vi "CRYUnflatten Work State.vi"(11 "Unflatten work state #":string) -> (0 "Error?":bool=TRUE, 3 "Header info":T1={"Data type"="Data            ", "Version"=1, "Dimensions"=0})   [LabVIEW 2013]
uses:
  CRYSystem/Hardware/CRYHardware Global.vi
  CRYSystem/Calibration/SubVI/CRYCal Global.vi
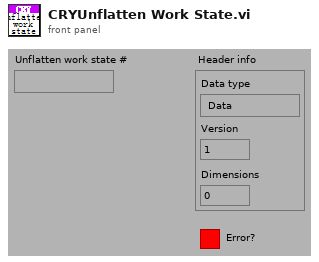
[diagram p1: front panel]
types:
  T1 = cluster{"Data type":string, "Version":u16, "Dimensions":u8}
  T2 = cluster{"unsigned byte array[0]":u8, "unsigned byte array[1]":u8, "unsigned byte array[2]":u8}
  T3 = cluster{"Mic Vol-L":dbl, "Mic Vol-R":dbl, "Mic Res-L":dbl, "Mic Res-R":dbl}
  T4 = cluster{"Mic Vol-L":dbl, "Mic Vol-R":dbl, "Mic Res-L":dbl, "Mic Res-R":dbl, "Mic Res-R 2":dbl, "Mic Res-R 3":dbl}
  T5 = cluster{"substring":string, u16, "unsigned byte array[2]":u8}
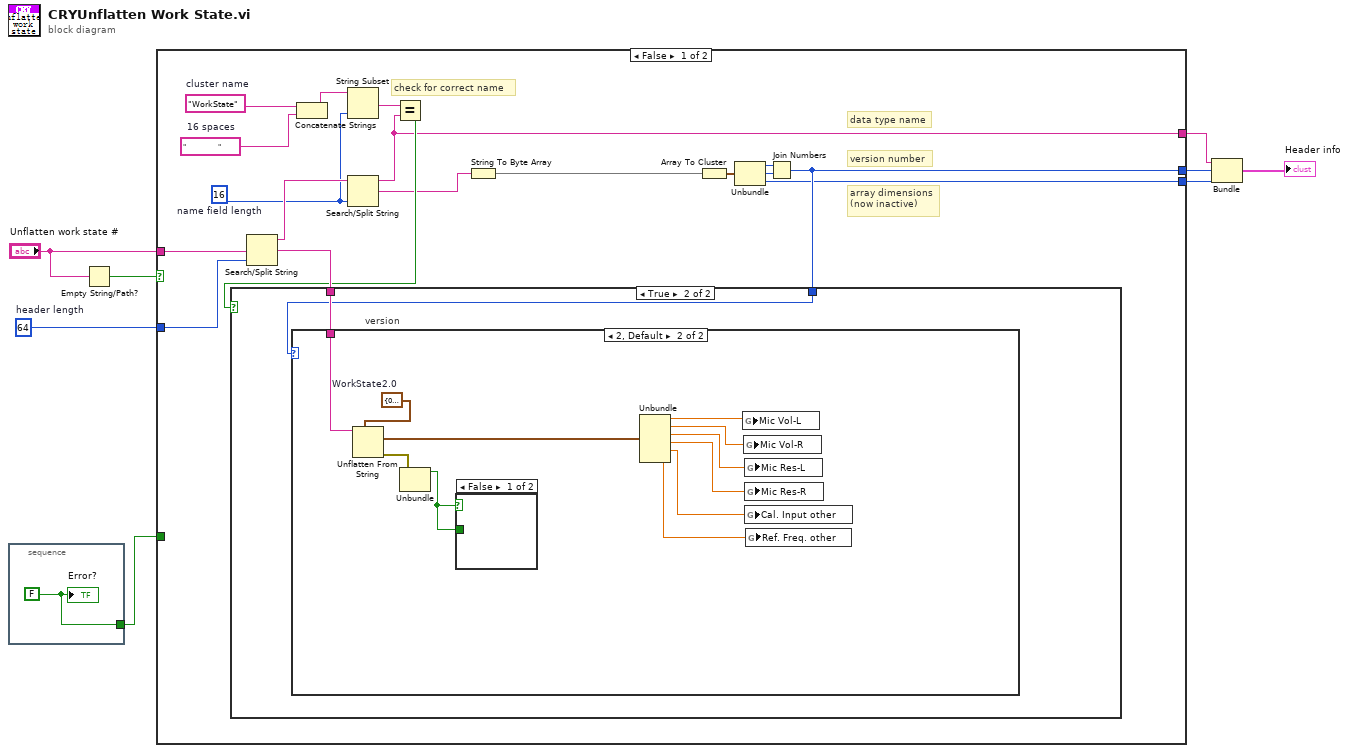
[diagram p0: block diagram]
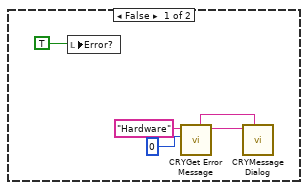
[diagram p2: hidden frame]
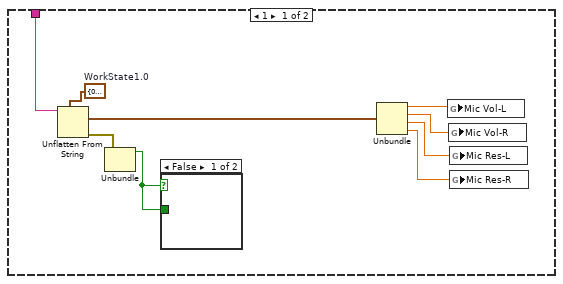
[diagram p3: hidden frame]
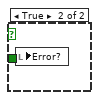
[diagram p4: hidden frame]
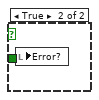
[diagram p5: hidden frame]
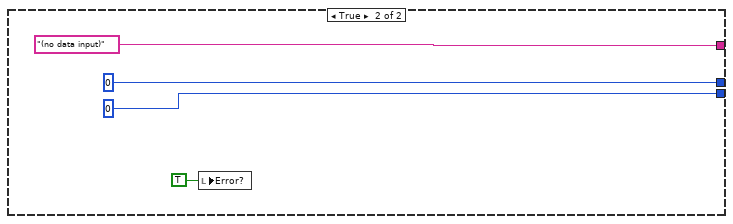
[diagram p6: hidden frame]
diagram:
  w5 = 64  # header length
  n1 = stacked-sequence {
    tunnel: [w9] -> w1
    frame #0 {
      w9 = FALSE
      "Error?" <- w9
    }
  }
  n2 = Empty String/Path?(string/path="Unflatten work state #") -> (empty?=w6:bool)
  n3 = case shown="False" w6 {
    tunnel: "Unflatten work state #" -> [w27 _]
    tunnel: w5 -> [w21 _]
    tunnel: [w18 u16 0] -> w3
    tunnel: [w10 u8 0] -> w4
    tunnel: [w11 "(no data input)" ("substring")] -> w2
    tunnel: w1 -> [_ _]
    frame False {
      w15 = "                "  # 16 spaces
      w16 = "WorkState"  # cluster name
      w13 = 16  # name field length
      # "check for correct name"
      # "array dimensions\n(now inactive)"
      # "version number"
      # "data type name"
      n4 = Search/Split String(string=w27, offset (0)=w21) -> (substring before match=w20:string, match + rest of string=w22:string)  [unwired: 2 out]
      n5 = Concatenate Strings(w16, w15) -> (w14:string)
      n6 = String Subset(string=w14, length (rest)=w13) -> (substring=w12:string)  [unwired: 1 out]
      n7 = Search/Split String(string=w20, offset (0)=w13) -> (substring before match=w11:string, match + rest of string=w17:string)  [unwired: 2 out]
      n8 = Equal?(x=w12, y=w11) -> (x = y?=w19:bool)
      n9 = String To Byte Array(string=w17) -> (unsigned byte array=w26:u8[])
      n10 = Array To Cluster(array=w26) -> (cluster=w25:T2)
      n11 = Unbundle(w25) -> ("unsigned byte array[0]"=w24:u8, "unsigned byte array[1]"=w23:u8, "unsigned byte array[2]"=w10:u8)
      n12 = Join Numbers(hi=w24, lo=w23) -> ((hi.lo)=w18:u16)
      n13 = case shown="True" w19 {
        tunnel: w22 -> [_ w34]
        tunnel: w18 -> [_ w33]
        frame False {
          n14 = local write "Error?"(TRUE) -> ()
          n15 = call "CRYGet Error Message.vi"("Error No"=0, "Kind"="Hardware") -> ("Message"=w29:string, "Window Title"=w28:string)  [unwired: 4 in, 4 out]
          n16 = call "CRYMessage Dialog.vi"("Window Title"=w28, "Message Content"=w29) -> ()  [unwired: 8 in, 2 out]
        }
        frame True {
          n17 = case "version" shown="2, Default" w33 {
            tunnel: w34 -> [w43 w55]
            frame 1 {
              w35 = T3 {"Mic Vol-L"=0.0, "Mic Vol-R"=0.0, "Mic Res-L"=0.0, "Mic Res-R"=0.0}  # WorkState1.0
              n18 = Unflatten From String(type=w35, binary string=w43) -> (value=w40:T3, error out=w41:errorcluster)  [unwired: 1 in, 3 out]
              n19 = Unbundle(w41) -> ("status"=w42:bool)  [unwired: 2 out]
              n20 = case shown="False" w42 {
                tunnel: w42 -> [_ w44]
                frame False {
                }
                frame True {
                  n21 = local write "Error?"(w44) -> ()
                }
              }
              n22 = Unbundle(w40) -> ("Mic Vol-L"=w39:dbl, "Mic Vol-R"=w38:dbl, "Mic Res-L"=w37:dbl, "Mic Res-R"=w36:dbl)
              n23 = global write "CRYHardware Global.vi" "Mic Vol-L"(w39) -> ()
              n24 = global write "CRYHardware Global.vi" "Mic Vol-R"(w38) -> ()
              n25 = global write "CRYHardware Global.vi" "Mic Res-L"(w37) -> ()
              n26 = global write "CRYHardware Global.vi" "Mic Res-R"(w36) -> ()
            }
            frame 2, Default {
              w47 = T4 {"Mic Vol-L"=0.0, "Mic Vol-R"=0.0, "Mic Res-L"=0.0, "Mic Res-R"=0.0, "Mic Res-R 2"=0.0, "Mic Res-R 3"=0.0}  # WorkState2.0
              n27 = Unflatten From String(type=w47, binary string=w55) -> (value=w52:T4, error out=w53:errorcluster)  [unwired: 1 in, 3 out]
              n28 = Unbundle(w53) -> ("status"=w54:bool)  [unwired: 2 out]
              n29 = case shown="False" w54 {
                tunnel: w54 -> [_ w56]
                frame False {
                }
                frame True {
                  n30 = local write "Error?"(w56) -> ()
                }
              }
              n31 = Unbundle(w52) -> ("Mic Vol-L"=w51:dbl, "Mic Vol-R"=w50:dbl, "Mic Res-L"=w49:dbl, "Mic Res-R"=w48:dbl, "Mic Res-R 2"=w46:dbl, "Mic Res-R 3"=w45:dbl)
              n32 = global write "CRYHardware Global.vi" "Mic Vol-L"(w51) -> ()
              n33 = global write "CRYHardware Global.vi" "Mic Vol-R"(w50) -> ()
              n34 = global write "CRYHardware Global.vi" "Mic Res-L"(w49) -> ()
              n35 = global write "CRYHardware Global.vi" "Mic Res-R"(w48) -> ()
              n36 = global write "CRYCal Global.vi" "Cal. Input other"(w46) -> ()
              n37 = global write "CRYCal Global.vi" "Ref. Freq. other"(w45) -> ()
            }
          }
        }
      }
    }
    frame True {
      n38 = local write "Error?"(TRUE ("Error?")) -> ()
    }
  }
  n39 = Bundle("substring"=w2, w3, "unsigned byte array[2]"=w4) -> (→"Header info":T5)  [unwired: 1 out]
